vi "FGV_SCREEN_2_graph_accumulative.vi"(7 "options":T1, 8 "error_in":errorcluster, 11 "input":variant) -> (0 "error_out":errorcluster)   [LabVIEW 2020]
uses:
  FGV_SCREEN_2_graph_accumulative.ctl
  <vilib>/Utility/miscctls.llb/LVAnnotationListTypeDef.ctl
  FGV_SCREEN_2_graph_accumulative_references.ctl
  FGV_SCREEN_2_graph_accumulative_all_info.ctl
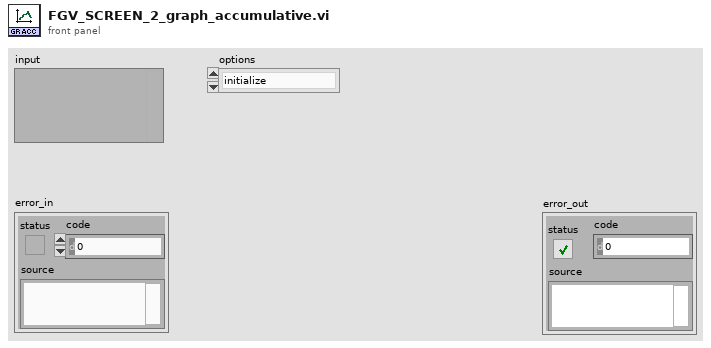
[diagram p1: front panel]
types:
  T1 = typedef "FGV_SCREEN_2_graph_accumulative.ctl" = enum16{"initialize", "set_hour_start", "set_hour_end", "set_target", "set_actual", "display"}
  T2 = typedef "FGV_SCREEN_2_graph_accumulative_all_info.ctl" = cluster{"hour_start":i8, "hour_end":i8, "actual_by_hour":u16[], "target_by_hour":u16[], "X_axis_labels":string[], "SCREEN_2_graph_accumulative_references":T3}
  T3 = typedef "FGV_SCREEN_2_graph_accumulative_references.ctl" = cluster{"graph_accumulative":refnum<vi>, "labels_picture_accumulative":refnum<vi>, "front_panel_reference":refnum<vi>}
  T4 = typedef "LVAnnotationListTypeDef.ctl" = cluster{"Name":string, "Color":u32, "Style":u8, "Point Style":u8, "Name Visible":bool, "Allow Drag":bool, "Annotation Mode":u32, "Plot":i32, "Index":i32, "Position":cluster{"X":dbl, "Y":dbl}, "X Scale":u32, "Y Scale":u32, "Show Arrow":bool, "Lock Name":bool, "Plot Area":i32, "Label Offset":cluster{"X":dbl, "Y":dbl}}[]
  T5 = cluster{"Name":string, "Color":u32, "Style":u8, "Point Style":u8, "Name Visible":bool, "Allow Drag":bool, "Annotation Mode":u32, "Plot":i32, "Index":i32, "Position":cluster{"X":dbl, "Y":dbl}, "X Scale":u32, "Y Scale":u32, "Show Arrow":bool, "Lock Name":bool, "Plot Area":i32, "Label Offset":cluster{"X":dbl, "Y":dbl}}[]
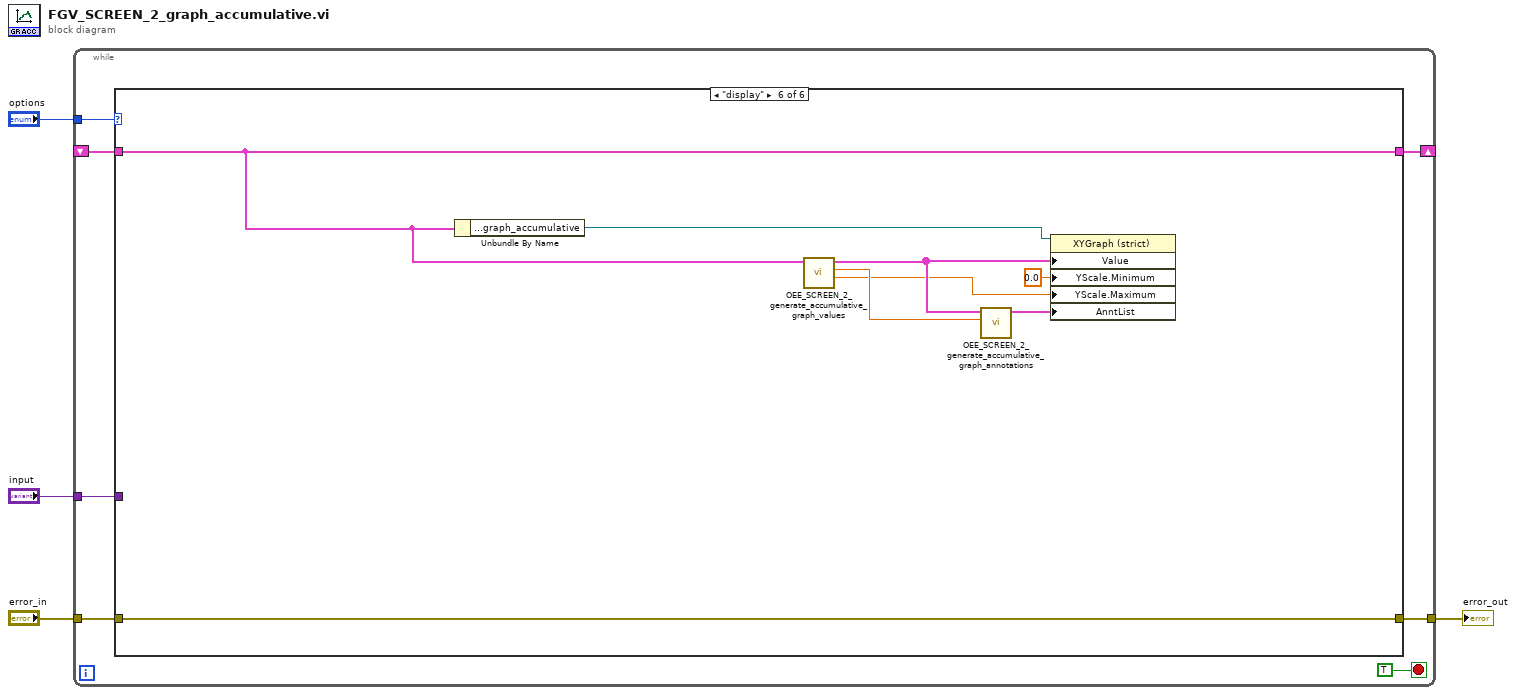
[diagram p0: block diagram]
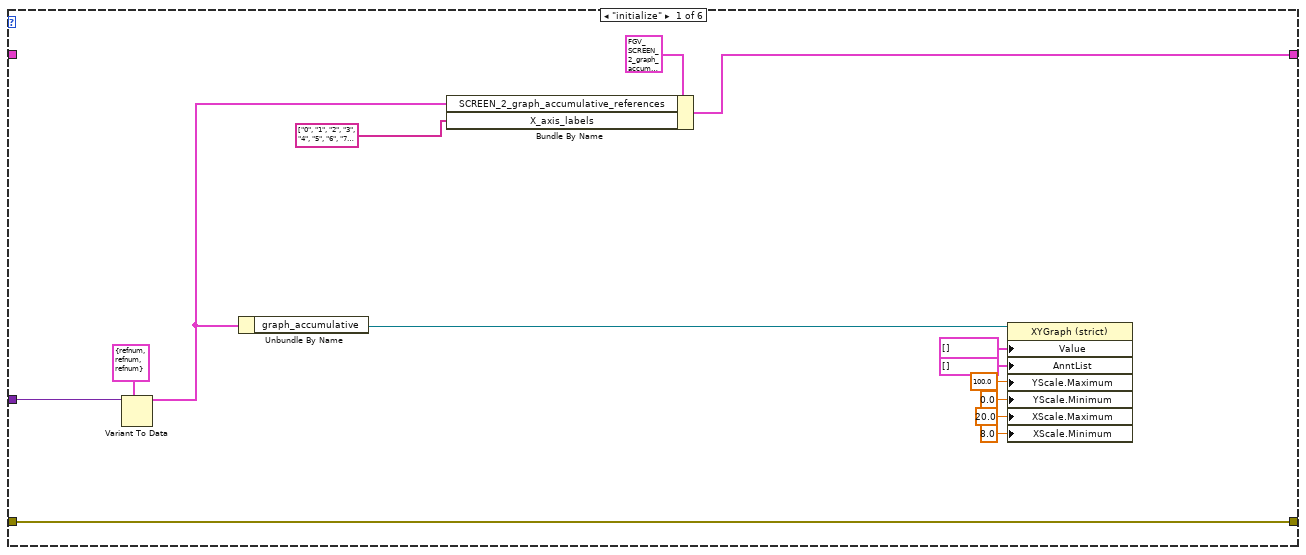
[diagram p2: hidden frame]
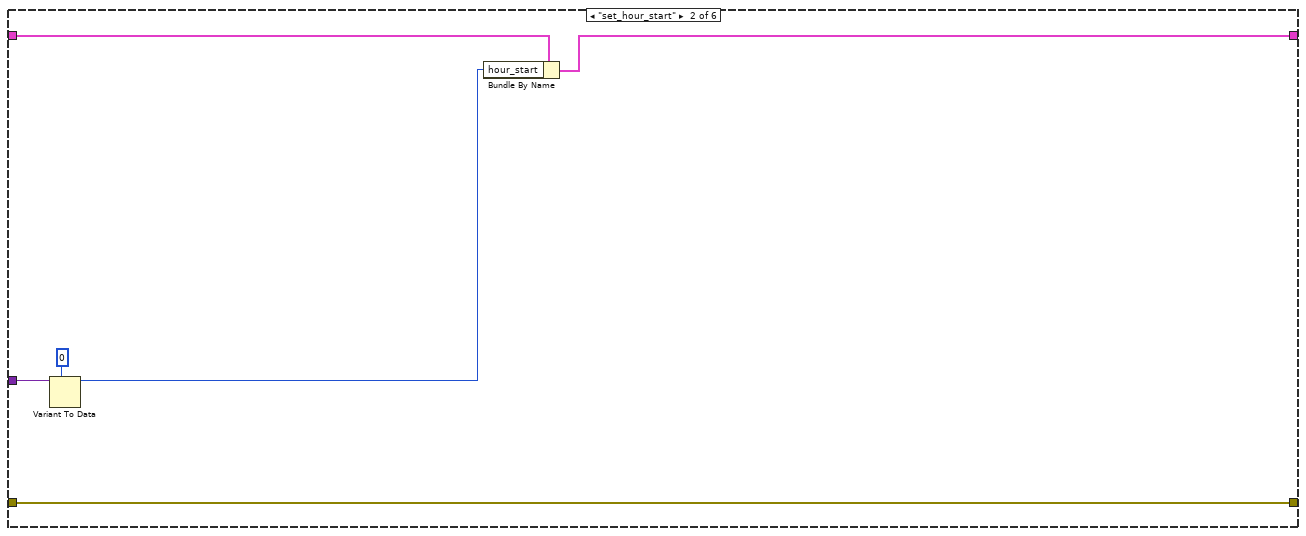
[diagram p3: hidden frame]
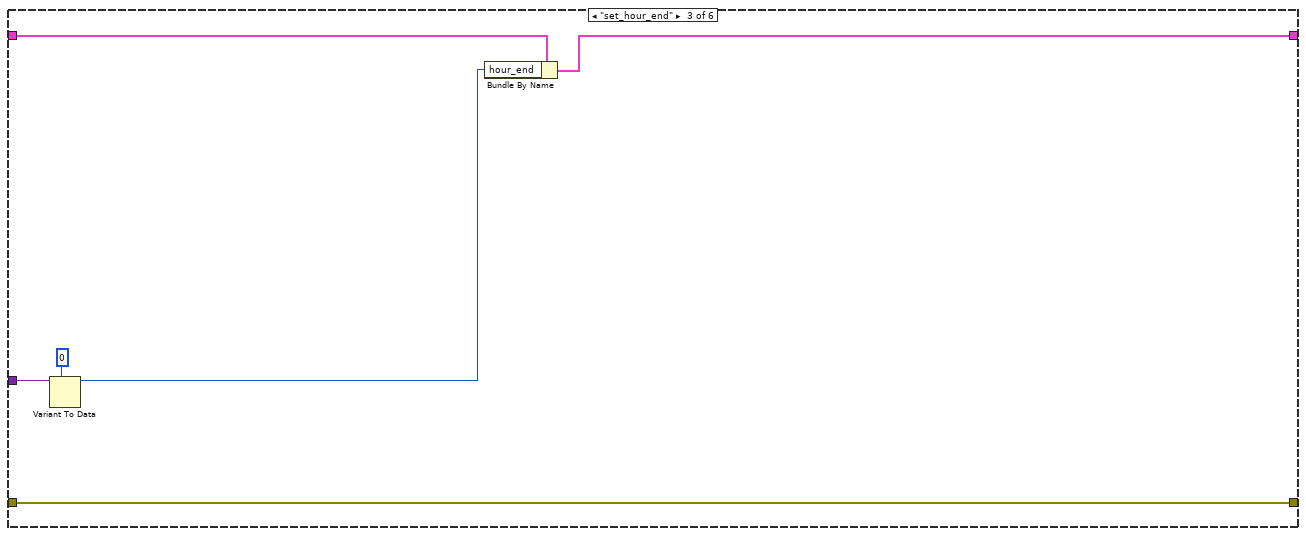
[diagram p4: hidden frame]
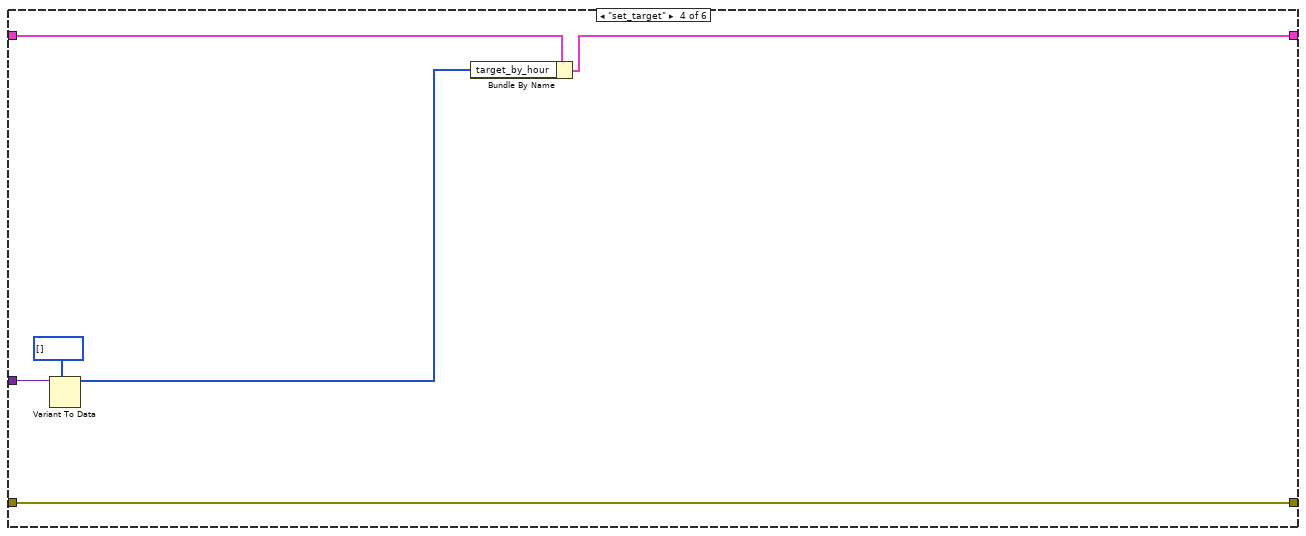
[diagram p5: hidden frame]
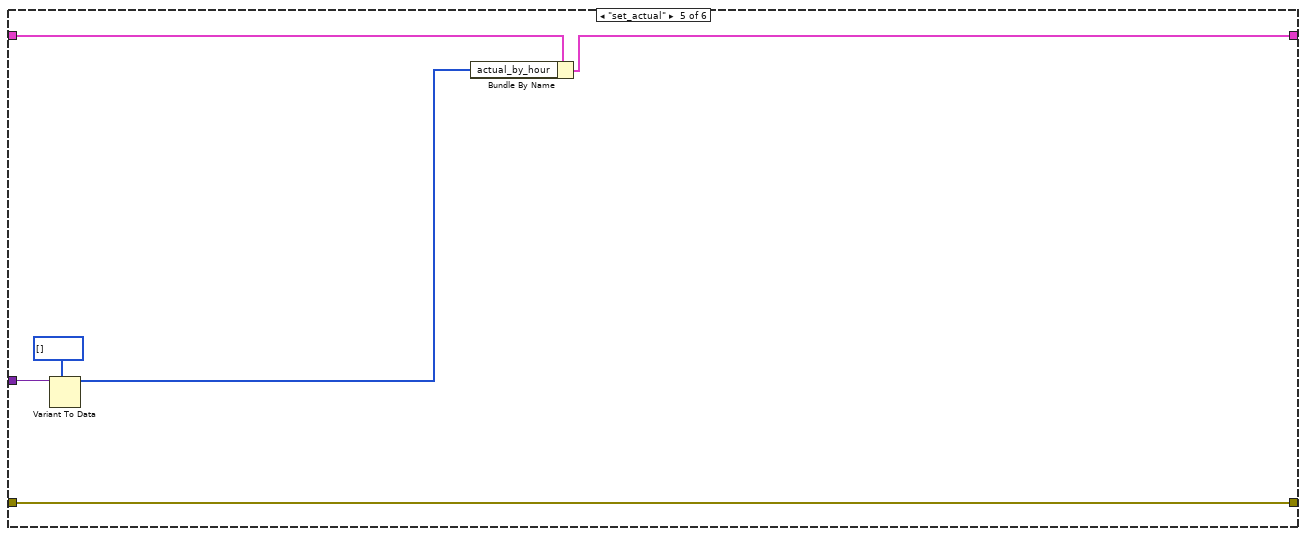
[diagram p6: hidden frame]
diagram:
  n1 = while {
    tunnel: "options" -> [w10]
    tunnel: [w9] -> w4
    tunnel: "error_in" -> [w8]
    shift-right: [w7] -> _
    shift-left: _ -> [w6]
    tunnel: "input" -> [w5]
    stop <- TRUE stop-if-true
    n2 = case shown="\"display\"" w10 {
      tunnel: [w25 w31 w37 w43 w49 w57] -> w9
      tunnel: w8 -> [w25 w31 w37 w43 w49 w57]
      tunnel: [w17 w26 w32 w40 w46 w51] -> w7
      tunnel: w6 -> [_ w28 w34 w41 w47 w51]
      tunnel: w5 -> [w16 w29 w35 w42 w48 _]
      frame "initialize" {
        n3 = Variant To Data(type=T3 {"graph_accumulative"=refnum, "labels_picture_accumulative"=refnum, "front_panel_reference"=refnum} ("OBJ_references"), Variant=w16) -> (data=w14:T3)  [unwired: 1 in, 1 out]
        n4 = Unbundle By Name(w14) -> ("graph_accumulative"=w13:refnum<vi>)
        n5 = Bundle By Name(cluster=T2 {"hour_start"=8, "hour_end"=8, "actual_by_hour"=[], "target_by_hour"=[], "X_axis_labels"=[], "SCREEN_2_graph_accumulative_references"={"graph_accumulative"=refnum, "labels_picture_accumulative"=refnum, "front_panel_reference"=refnum}} ("SCREEN_2_graph_accumulative_all_info"), "SCREEN_2_graph_accumulative_references"=w14, "X_axis_labels"=string[] ["0", "1", "2", "3", "4", "5", "6", "7", "8", "9", "10", "11", "12", "13", "14", "15", "16", "17", "18", "19", "20", "21", "22", "23"]) -> (w17:T2)
        n6 = property class="XYGraph (strict)"(reference=w13, "Value"=cluster{dbl[], dbl[]}[] [], "AnntList"=T4 [] ("Annotation List"), "YScale.Maximum"=100.0 ("Y Scale.Range:Maximum"), "YScale.Minimum"=0.0 ("Y Scale.Range:Minimum"), "XScale.Maximum"=20.0 ("X Scale.Range:Maximum"), "XScale.Minimum"=8.0 ("X Scale.Range:Minimum")) -> ()  [unwired: 1 in, 2 out]
      }
      frame "set_hour_start" {
        n7 = Variant To Data(type=i8 0 ("hour_start"), Variant=w29) -> (data=w27:i8)  [unwired: 1 in, 1 out]
        n8 = Bundle By Name(cluster=w28, "hour_start"=w27) -> (w26:T2)
      }
      frame "set_hour_end" {
        n9 = Variant To Data(type=i8 0 ("hour_start"), Variant=w35) -> (data=w33:i8)  [unwired: 1 in, 1 out]
        n10 = Bundle By Name(cluster=w34, "hour_end"=w33) -> (w32:T2)
      }
      frame "set_target" {
        n11 = Variant To Data(type=u16[] [] ("actual_by_hour"), Variant=w42) -> (data=w38:u16[])  [unwired: 1 in, 1 out]
        n12 = Bundle By Name(cluster=w41, "target_by_hour"=w38) -> (w40:T2)
      }
      frame "set_actual" {
        n13 = Variant To Data(type=u16[] [] ("actual_by_hour"), Variant=w48) -> (data=w44:u16[])  [unwired: 1 in, 1 out]
        n14 = Bundle By Name(cluster=w47, "actual_by_hour"=w44) -> (w46:T2)
      }
      frame "display" {
        n15 = Unbundle By Name(w51) -> ("SCREEN_2_graph_accumulative_references.graph_accumulative"=w52:refnum<vi>)
        n16 = call "OEE_SCREEN_2_generate_accumulative_graph_values.vi"("SCREEN_2_graph_accumulative_all_info"=w51) -> ("Y_scale_max"=w54:dbl, "Y_annotation_offset"=w55:dbl, "graph_values"=w56:cluster{dbl[], dbl[]}[])  [unwired: 8 in]
        n17 = call "OEE_SCREEN_2_generate_accumulative_graph_annotations.vi"("Y_annotation_offset"=w55, "graph_values"=w56) -> ("Array"=w53:T5)  [unwired: 9 in]
        n18 = property class="XYGraph (strict)"(reference=w52, "Value"=w56, "YScale.Minimum"=0.0 ("Y Scale.Range:Minimum"), "YScale.Maximum"=w54, "AnntList"=w53) -> ()  [unwired: 1 in, 2 out]
      }
    }
  }
  "error_out" <- w4
